vi "Set RON and return RON status.vi"(0 "System no.":i32=1 min=1 max=4 step=1, 2 "Affected axes":string[](array[string]), 3 "All axes?":bool, 4 "Reference mode":bool[](array[boolean]), 5 "error in":errorcluster) -> (14 "Axes with RON OFF":string[](array[string]), 15 "Axes with RON ON":string[](array[string]), 19 "error out":errorcluster)   [LabVIEW 2020]
doc: "Sets RON mode ON or OFF and returns which of the connected axes have RON mode ON and which have RON mode OFF. \nIf reference mode is OFF, no referencing is required for the axis. Only relative moves can be commanded (using MVR.vi), unless the actual position is set with POS.vi. Afterwards, relative and absolute moves can be commanded.\nFor stages with neither reference nor limit switch, reference mode is automatically OFF. \nWARNING! If reference mode is switched off, and relative moves are commanded, stages can be driven into the mechanical hard stop if moving to a position which is outside the travel range! \nIf reference mode is switched off, and the actual position is incorrectly set with POS.vi, stages can be driven into the mechanical hard stop when moving to a position which is thought to be within the travel range of the stage, but actually is not."
panel:
  # "Sets RON mode ON or OFF and returns which of the connected axes have RON mode ON and which have \nRON mode OFF. \nIf reference mode is OFF, no referencing is required for the axis. Only relative moves can be commanded (using \n\"MVR.vi\"), unless the actual position is set with POS.vi. Afterwards, relative and absolute moves can be commanded.\nFor stages with neither reference nor limit switch, reference mode is automatically OFF. \n\nWARNING! If reference mode is switched off, and relative movements are commanded, stages can be \ndriven into the mechanical hard stop if moving to a position which is outside the travel range! \nIf reference mode is switched off, and the actual position is incorrectly set with \"POS.vi\", stages can be \ndriven into the mechanical hard stop when moving to a position which is thought to be within the travel \nrange of the stage, but actually is not."
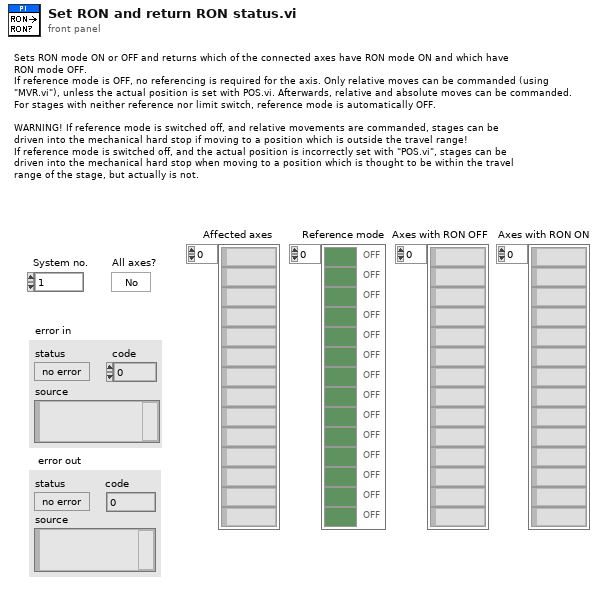
[diagram p1: front panel]
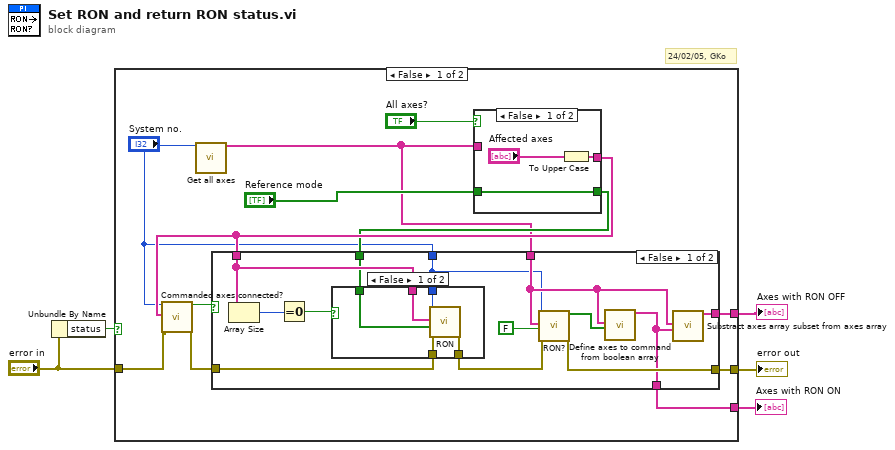
[diagram p0: block diagram]
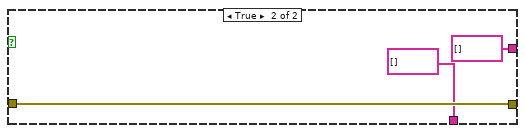
[diagram p3: hidden frame]
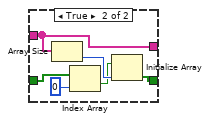
[diagram p4: hidden frame]
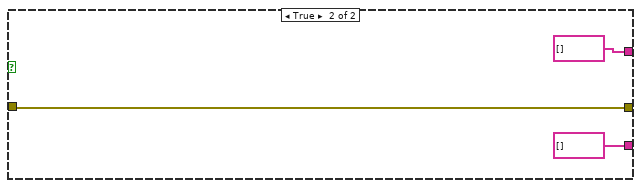
[diagram p5: hidden frame]
diagram:
  # "24/02/05, GKo"
  n1 = Unbundle By Name("error in") -> ("status"=w1:bool)
  n2 = case shown="False" w1 {
    tunnel: [w17 w50] -> w5
    tunnel: [w15 string[] [] ("Axes to command")] -> w4
    tunnel: [w14 string[] [] ("Axes to command")] -> w3
    tunnel: "error in" -> [w11 w50]
    frame False {
      n3 = call "Get all axes.vi"("System no."="System no.") -> ("Conn. Axes"=w6:string[])  [unwired: 18 out]
      n4 = case shown="False" "All axes?" {
        tunnel: [w41 w48] -> w13
        tunnel: w6 -> [_ w48]
        tunnel: [w40 w43] -> w9
        tunnel: "Reference mode" -> [w40 w47]
        frame False {
          n5 = To Upper Case(1:"Affected axes") -> (0:w41:string[])
        }
        frame True {
          n6 = Array Size(array=w48) -> (size(s)=w45:i32)
          n7 = Index Array(array=w47, index=0 ("Index")) -> (element=w44:bool)
          n8 = Initialize Array(w44, w45) -> (w43:bool[])
        }
      }
      n9 = call "Commanded axes connected?.vi"("System no."="System no.", "Commanded axes"=w13, "error in"=w11) -> ("Controller error"=w10:bool, "error out"=w12:errorcluster)  [unwired: 15 out]
      n10 = case shown="False" w10 {
        tunnel: [w30 w39] -> w17
        tunnel: w6 -> [w29 _]
        tunnel: [w28 string[] [] ("Axes to command")] -> w15
        tunnel: [w27 string[] [] ("Axes to command")] -> w14
        tunnel: "System no." -> [w23 _]
        tunnel: w13 -> [w22 _]
        tunnel: w12 -> [w21 w39]
        tunnel: w9 -> [w18 _]
        frame False {
          n11 = Array Size(array=w22) -> (size(s)=w19:i32)
          n12 = Equal To 0?(x=w19) -> (x = 0?=w20:bool)
          n13 = case shown="False" w20 {
            tunnel: [w35 w36] -> w24
            tunnel: w23 -> [w34 _]
            tunnel: w22 -> [w33 _]
            tunnel: w21 -> [w32 w36]
            tunnel: w18 -> [w31 _]
            frame False {
              n14 = call "RON.vi"("System no."=w34, "Axes to command"=w33, "Reference mode"=w31, "error in"=w32) -> ("error out"=w35:errorcluster)  [unwired: 1 in, 14 out]
            }
            frame True {
            }
          }
          n15 = call "RON?.vi"("System no."=w23, "Axes to query"=w29, "All axes?"=FALSE, "error in"=w24) -> ("Reference on?"=w26:bool[], "error out"=w30:errorcluster)  [unwired: 1 in, 13 out]
          n16 = call "Define axes to command from boolean array.vi"("Axes to query"=w29, "Command axis?"=w26) -> ("Axes to command"=w27:string[])  [unwired: 4 in, 13 out]
          n17 = call "Substract axes array subset from axes array.vi"("Axes to query"=w29, "Axes subset"=w27) -> ("Axes to command"=w28:string[])  [unwired: 1 in, 16 out]
        }
        frame True {
        }
      }
    }
    frame True {
    }
  }
  "error out" <- w5
  "Axes with RON OFF" <- w4
  "Axes with RON ON" <- w3
